vi "the effect capacity fading RT.vi"(4 "Cycling\ntemperature\nto K factors":u16, 5 "N cycles":dbl, 6 "Time cell\nnot used(months)":dbl, 7 "temperature(ªC) battery not used":dbl, 8 "capacity cell":dbl) -> (0 "R cycle":dbl, 1 "cycle life losses(%)":dbl, 2 "calendar life losses(%)":dbl, 3 "capacity usable(Ah)":dbl)   [LabVIEW 2017]
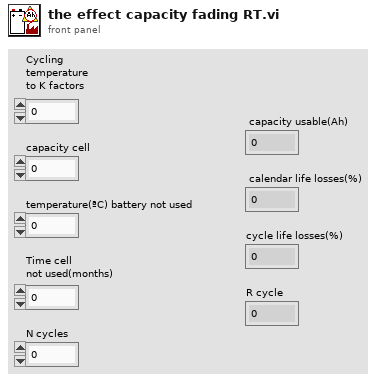
[diagram p1: front panel]
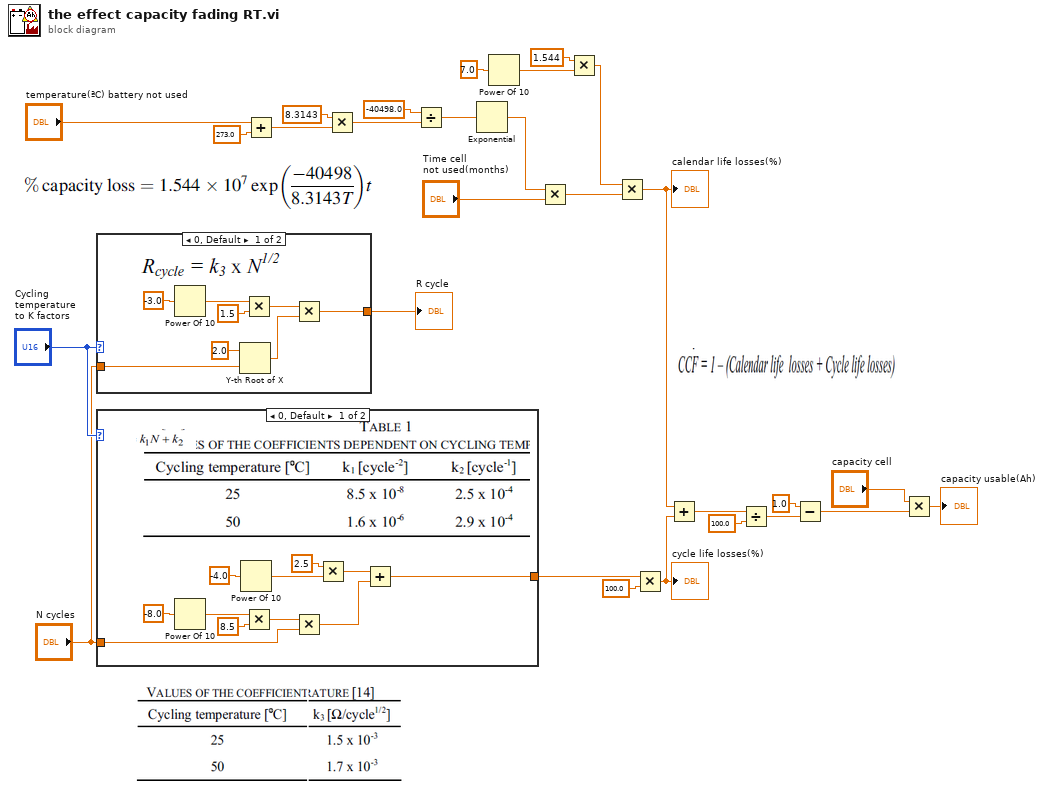
[diagram p0: block diagram]
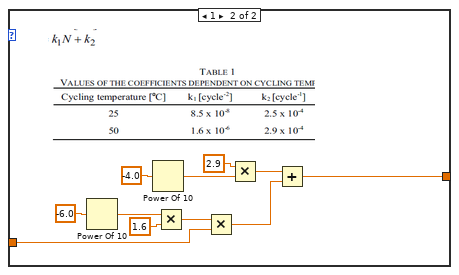
[diagram p2: hidden frame]
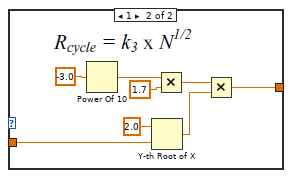
[diagram p3: hidden frame]
diagram:
  n1 = case shown="0, Default" "Cycling\ntemperature\nto K factors" {
    tunnel: "N cycles" -> [w35 w38]
    tunnel: [w29 w37] -> w9
    frame 0, Default {
      n2 = Power Of 10(x=-3.0) -> (10^x=w32:dbl)
      n3 = Y-th Root of X(1:w35, 2:2.0 ("y")) -> (0:w34:dbl)
      n4 = Multiply(x=w32, y=1.5) -> (x*y=w30:dbl)
      n5 = Multiply(x=w30, y=w34) -> (x*y=w29:dbl)
    }
    frame 1 {
      n6 = Power Of 10(x=-3.0) -> (10^x=w41:dbl)
      n7 = Y-th Root of X(1:w38, 2:2.0 ("y")) -> (0:w43:dbl)
      n8 = Multiply(x=w41, y=1.7) -> (x*y=w39:dbl)
      n9 = Multiply(x=w39, y=w43) -> (x*y=w37:dbl)
    }
  }
  "R cycle" <- w9
  n10 = case shown="0, Default" "Cycling\ntemperature\nto K factors" {
    tunnel: [w45 w57] -> w11
    tunnel: "N cycles" -> [w46 w56]
    frame 0, Default {
      n11 = Power Of 10(x=-8.0) -> (10^x=w50:dbl)
      n12 = Power Of 10(x=-4.0) -> (10^x=w49:dbl)
      n13 = Multiply(x=w50, y=8.5) -> (x*y=w52:dbl)
      n14 = Multiply(x=w52, y=w46) -> (x*y=w55:dbl)
      n15 = Multiply(x=2.5, y=w49) -> (x*y=w47:dbl)
      n16 = Add(x=w47, y=w55) -> (x+y=w45:dbl)
    }
    frame 1 {
      n17 = Power Of 10(x=-6.0) -> (10^x=w61:dbl)
      n18 = Power Of 10(x=-4.0) -> (10^x=w60:dbl)
      n19 = Multiply(x=w61, y=1.6) -> (x*y=w63:dbl)
      n20 = Multiply(x=w63, y=w56) -> (x*y=w66:dbl)
      n21 = Multiply(x=2.9, y=w60) -> (x*y=w58:dbl)
      n22 = Add(x=w58, y=w66) -> (x+y=w57:dbl)
    }
  }
  n23 = Add(x="temperature(ªC) battery not used", y=273.0) -> (x+y=w22:dbl)
  n24 = Multiply(x=8.3143, y=w22) -> (x*y=w17:dbl)
  n25 = Divide(x=-40498.0, y=w17) -> (x/y=w19:dbl)
  n26 = Exponential(1:w19) -> (0:w20:dbl)
  n27 = Power Of 10(x=7.0) -> (10^x=w13:dbl)
  n28 = Multiply(x=w20, y="Time cell\nnot used(months)") -> (x*y=w21:dbl)
  n29 = Multiply(x=1.544, y=w13) -> (x*y=w14:dbl)
  n30 = Multiply(x=w14, y=w21) -> (x*y=w4:dbl)
  "calendar life losses(%)" <- w4
  n31 = Multiply(x=w11, y=100.0) -> (x*y=w1:dbl)
  "cycle life losses(%)" <- w1
  n32 = Add(x=w4, y=w1) -> (x+y=w6:dbl)
  n33 = Divide(x=w6, y=100.0) -> (x/y=w8:dbl)
  n34 = Subtract(x=1.0, y=w8) -> (x-y=w28:dbl)
  n35 = Multiply(x="capacity cell", y=w28) -> (x*y=→"capacity usable(Ah)":dbl)
